vi "SendReceiveRAW.vi"(0 "connection ID":refnum<k16>, 1 "address":u32, 2 "port":u16, 5 "RAW data in":string="SR", 7 "Number of retries (3)":u8=3, 9 "timeout ms (1000)":i32=100, 11 "error in (no error)":errorcluster) -> (4 "connection ID out":refnum<k16>, 6 "received data":string, 15 "error out":errorcluster)   [LabVIEW 2016, in "instr.lvlib"]
doc: "Low level send and receive with multiple trials on timeout.\nAs UDP communication may fail, this is a soft approach to retry a few times before exiting with error."
uses:
  instr.lvlib
panel:
  out "Number of retries":i32
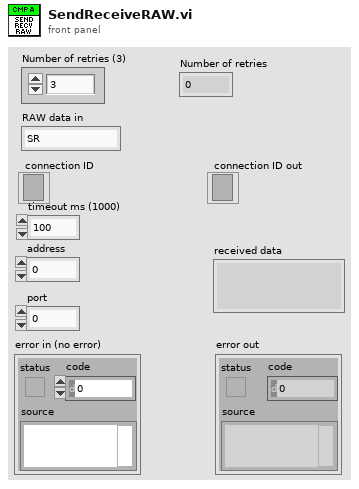
[diagram p1: front panel]
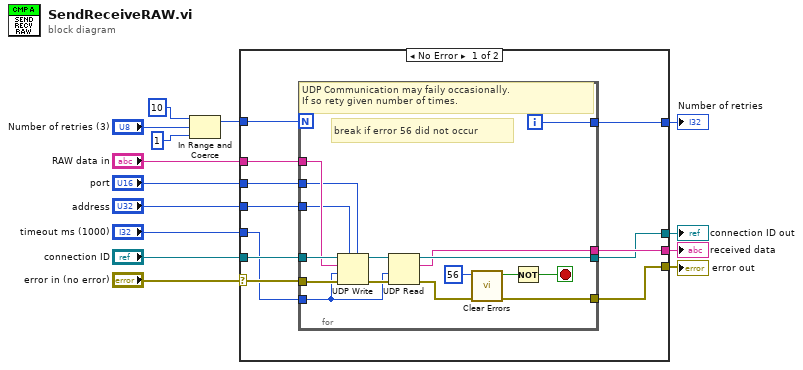
[diagram p0: block diagram]
diagram:
  n1 = In Range and Coerce(upper limit=u8 10, x="Number of retries (3)", lower limit=u8 1) -> (coerced(x)=w2:u8)  [unwired: 1 out]
  n2 = case shown="No Error" "error in (no error)" {
    selector: "error in (no error)" -> [w25 w43]
    tunnel: [w17 w43] -> w14
    tunnel: [w19 _] -> w12
    tunnel: "timeout ms (1000)" -> [w22 _]
    tunnel: "connection ID" -> [w24 w42]
    tunnel: [w18 w42] -> w9
    tunnel: "address" -> [w21 _]
    tunnel: "port" -> [w20 _]
    tunnel: "RAW data in" -> [w23 _]
    tunnel: w2 -> [w16 _]
    tunnel: [w15 _] -> w1
    frame No Error {
      n3 = for {
        N: w16 -> [_]
        tunnel: [w39] -> w15
        tunnel: [w41] -> w17
        tunnel: w25 -> [w34]
        tunnel: [w32] -> w18
        tunnel: w24 -> [w31]
        tunnel: w23 -> [w30]
        tunnel: w22 -> [w27]
        tunnel: w21 -> [w29]
        tunnel: w20 -> [w28]
        tunnel: [w26] -> w19
        i -> [w39]
        stop <- w38 stop-if-true
        # "break if error 56 did not occur"
        # "UDP Communication may faily occasionally. \nIf so rety given number of times."
        n4 = UDP Write(address=w29, port or service name=w28, connection ID=w31, data in=w30, 8:w34, 9:w27) -> (error out=w36:errorcluster, 3:w35:refnum<k16>)
        n5 = UDP Read(connection ID=w35, timeout ms (25000)=w27, 8:w36) -> (data out=w26:string, error out=w33:errorcluster, 3:w32:refnum<k16>)  [unwired: 1 in, 2 out]
        n6 = call <vilib>:"Clear Errors.vi"("error in (no error)"=w33, "specific error code to clear (0: all)"=56) -> ("error out"=w41:errorcluster, "specific error cleared?"=w37:bool)  [unwired: 4 in]
        n7 = Not(x=w37) -> (.not. x?=w38:bool)
      }
    }
    frame Error {
    }
  }
  "error out" <- w14
  "received data" <- w12
  "connection ID out" <- w9
  "Number of retries" <- w1
